vi "写入单个线圈.vi"(8 "error in":errorcluster, 10 "写入线圈信息组":cluster{"地址":u16, "布尔":bool, "名称":string}[](array[cluster]), 11 "MB_实体":refnum<class "Modbus Master.lvclass">) -> (0 "输出簇":errorcluster, 3 "连接成功":bool)   [LabVIEW 2015]
uses:
  <vilib>/NI/Modbus Library/API/Master/Modbus Master.lvclass
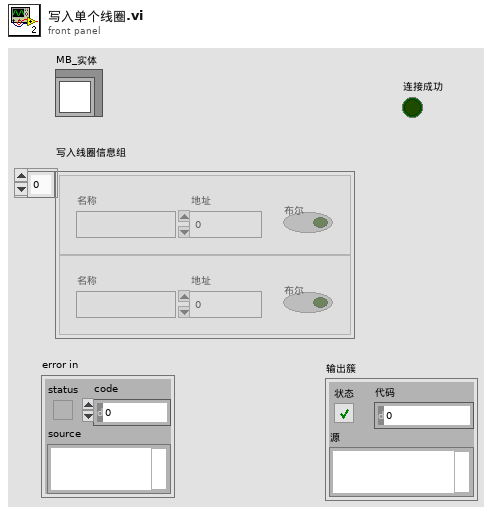
[diagram p1: front panel]
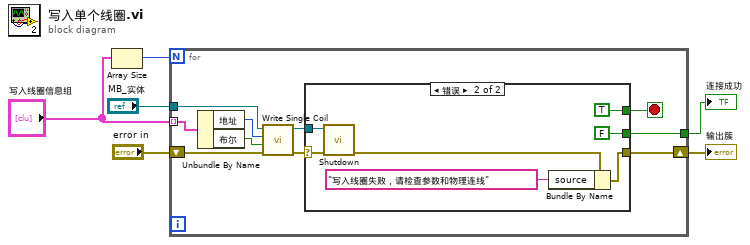
[diagram p0: block diagram]
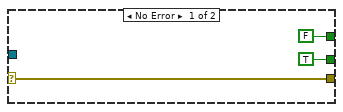
[diagram p2: hidden frame]
diagram:
  n1 = Array Size(array="写入线圈信息组") -> (size(s)=w5:i32)
  n2 = for {
    N: w5 -> [_]
    tunnel: [w16] -> w4
    tunnel: "MB_实体" -> [w12]
    shift-right: [w10] -> w2
    shift-left: "error in" -> [w11]
    tunnel: "写入线圈信息组" -> [w9] mode=indexing
    stop <- w15 stop-if-true
    n3 = Unbundle By Name(w9) -> ("地址"=w8:u16, "布尔"=w7:bool)
    n4 = call-dynamic "Write Single Coil.vi"("error in"=w11, "coil to write"=w7, "address"=w8, "Modbus master in"=w12) -> ("error out"=w14:errorcluster, "Modbus master out"=w13:refnum<class "Modbus Master.lvclass">)  [unwired: 6 in]
    n5 = case shown="错误" w14 {
      selector: w14 -> [w18 w24]
      tunnel: [TRUE FALSE] -> w16
      tunnel: [FALSE TRUE] -> w15
      tunnel: w13 -> [_ w23]
      tunnel: [w18 w20] -> w10
      frame No Error {
      }
      frame Error {
        n6 = call-dynamic "Shutdown.vi"("error in"=w24, "Modbus master in"=w23) -> ("error out"=w22:errorcluster)  [unwired: 9 in]
        n7 = Bundle By Name(cluster=w22, "source"="写入线圈失败，请检查参数和物理连线" ("消息")) -> (w20:errorcluster)
      }
    }
  }
  "连接成功" <- w4
  "输出簇" <- w2
